vi "FW Set Position.vi"(0 "Notifier Name In":string, 2 "Wait for Finish":bool=TRUE, 7 "Position":i32, 11 "Error In":errorcluster) -> (4 "Notifier Name Out":string, 15 "Error Out":errorcluster)   [LabVIEW 2020]
uses:
  FW Type Defs/FW Notifier Type.ctl
  FW Type Defs/FW Actions.ctl
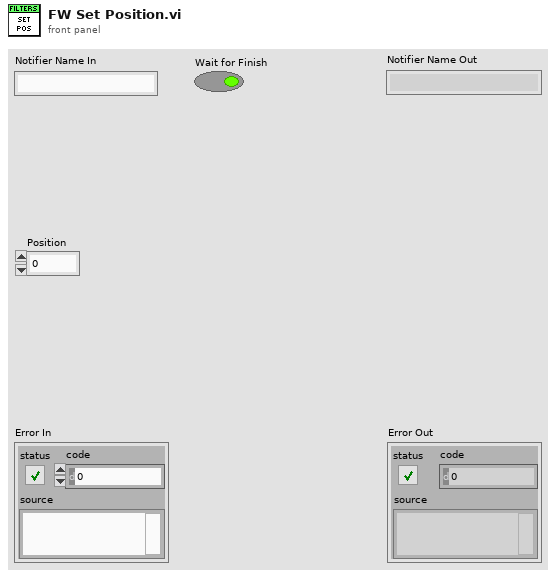
[diagram p1: front panel]
types:
  T1 = typedef "FW Notifier Type.ctl" = cluster{"Actions":T2, "Set Position":u8, "Actual Position":u8, "Speed":dbl, "Num Positions":u8, "Received":bool}
  T2 = typedef "FW Actions.ctl" = enum16{"Set Position", "Get Position", "Get Num Positions", "Set Speed", "Confirm Pos", "Quit"}
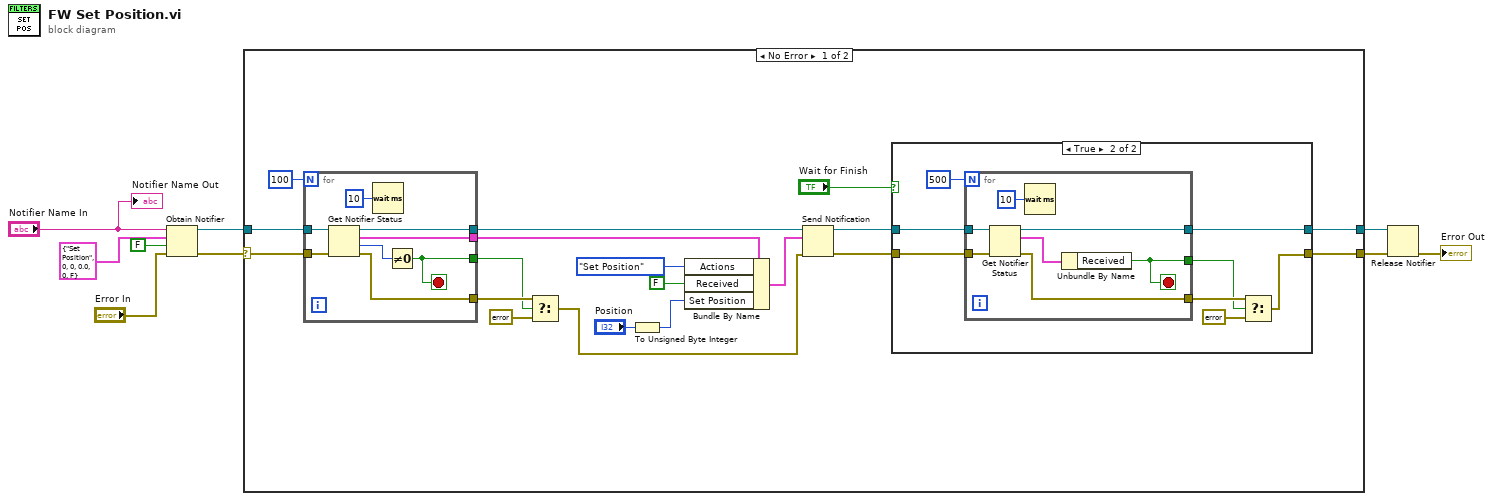
[diagram p0: block diagram]
diagram:
  n1 = Obtain Notifier(name (unnamed)="Notifier Name In", notification data type=T1 {"Actions"=enum."Set Position", "Set Position"=0, "Actual Position"=0, "Speed"=0.0, "Num Positions"=0, "Received"=FALSE} ("FW102C Note Type"), create if not found? (T)=FALSE, error in (no error)="Error In") -> (notifier out=w6:refnum<notifier>, error out=w7:errorcluster)  [unwired: 1 out]
  n2 = case shown="No Error" w7 {
    selector: w7 -> [w26 w55]
    tunnel: w6 -> [w28 w54]
    tunnel: [w20 w55] -> w3
    tunnel: [w21 w54] -> w4
    frame No Error {
      n3 = for {
        N: 100 -> [_]
        tunnel: w28 -> [w53]
        tunnel: [w51] -> w17
        tunnel: [w49] -> w25
        tunnel: w26 -> [w48]
        tunnel: [w47] -> w18
        tunnel: [w46] -> w13
        stop <- w51 stop-if-true
        n4 = Get Notifier Status(notifier=w53, error in (no error)=w48) -> (notifier out=w49:refnum<notifier>, current notification=w46:T1, # waiting=w52:i32, error out=w47:errorcluster)  [unwired: 1 out]
        n5 = Wait (ms)(milliseconds to wait=u32 10) -> ()  [unwired: 1 out]
        n6 = Not Equal To 0?(x=w52) -> (x != 0?=w51:bool)
      }
      n7 = Select(t=w18, s=w17, f=errorcluster {"status"=TRUE, "code"=0, "source"="Filter wheel busy. Timeout error."}) -> (s? t:f=w12:errorcluster)
      n8 = To Unsigned Byte Integer(number="Position") -> (unsigned 8bit integer=w10:u8)
      n9 = Bundle By Name(cluster=w13, "Actions"=FW_Actions."Set Position", "Received"=FALSE, "Set Position"=w10) -> (w24:T1)
      n10 = Send Notification(notification=w24, notifier=w25, error in (no error)=w12) -> (notifier out=w22:refnum<notifier>, error out=w23:errorcluster)
      n11 = case shown="True" "Wait for Finish" {
        tunnel: w23 -> [w29 w38]
        tunnel: w22 -> [w30 w37]
        tunnel: [w30 w36] -> w21
        tunnel: [w29 w35] -> w20
        frame False {
        }
        frame True {
          n12 = for {
            N: 500 -> [_]
            tunnel: w37 -> [w45]
            tunnel: [w43] -> w36
            tunnel: w38 -> [w42]
            tunnel: [w41] -> w33
            tunnel: [w39] -> w32
            stop <- w39 stop-if-true
            n13 = Get Notifier Status(notifier=w45, error in (no error)=w42) -> (notifier out=w43:refnum<notifier>, current notification=w40:T1, error out=w41:errorcluster)  [unwired: 2 out]
            n14 = Wait (ms)(milliseconds to wait=u32 10) -> ()  [unwired: 1 out]
            n15 = Unbundle By Name(w40) -> ("Received"=w39:bool)
          }
          n16 = Select(t=w33, s=w32, f=errorcluster {"status"=TRUE, "code"=0, "source"="Filter Wheel Error: Action didn't complete."}) -> (s? t:f=w35:errorcluster)
        }
      }
    }
    frame Error {
    }
  }
  n17 = Release Notifier(notifier=w4, error in (no error)=w3) -> (error out=→"Error Out":errorcluster)  [unwired: 1 in, 2 out]
  "Notifier Name Out" <- "Notifier Name In"
